vi "heterochromaticFlicker_digitalIN.vi"() -> ()   [LabVIEW 2011]
uses:
  <vilib>/LabVIEW Interface for Arduino/Type Defs/Pin Mode.ctl
  <vilib>/LabVIEW Interface for Arduino/LabVIEW Interface for Arduino.lvlib
panel:
  out "BUTTON":bool
  out "Joy DOWN":bool
  out "Joy UP":bool
  in  "Button Pin":u8=2
  in  "Joy DOWN Pin":u8=2
  in  "Joy UP Pin":u8=2
  in  "Stop":bool
  out "Debug \ninner i\n(which of the\nlights to be flashed)":i32
  out "Debug \nouter i\n(how many \ncycles passed)":i32
  in  "Duty Cycle 410nm 3":u8(slide) step=1 scale=0.0..255.0
  in  "Pin 560nm":dbl=2.0
  in  "Pin 410nm":dbl=2.0
  out "Flicker period [ms]":dbl=500.0
  in  "Flicker Freq [Hz]":dbl=2.0 min=0.2 max=100.0 step=0.1
  in  "Duty Cycle 410nm":u8(slide) step=1 scale=0.0..255.0
  in  "Duty Cycle 560nm":u8(slide) step=1 scale=0.0..255.0
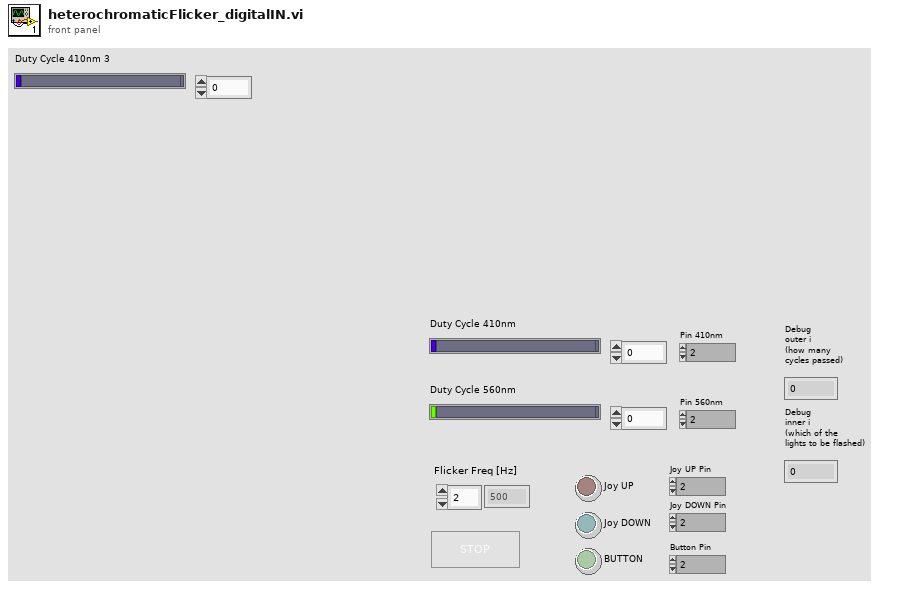
[diagram p1: front panel]
types:
  T1 = typedef "LabVIEW Interface for Arduino.lvlib/Arduino Resource.ctl" = cluster{"VISA resource":refnum<visa-resource-name>, "Board Type":T2, "Connection Type":enum8{"USB / Serial"}, "Bytes Per Packet (15)":u8}
  T2 = typedef "LabVIEW Interface for Arduino.lvlib/Board Type.ctl" = enum16{"Uno", "Dimuelanove w/Atmega 328", "Mega 2560"}
  T3 = typedef "LabVIEW Interface for Arduino.lvlib/Pin Mode.ctl" = enum8{"Input", "Output"}
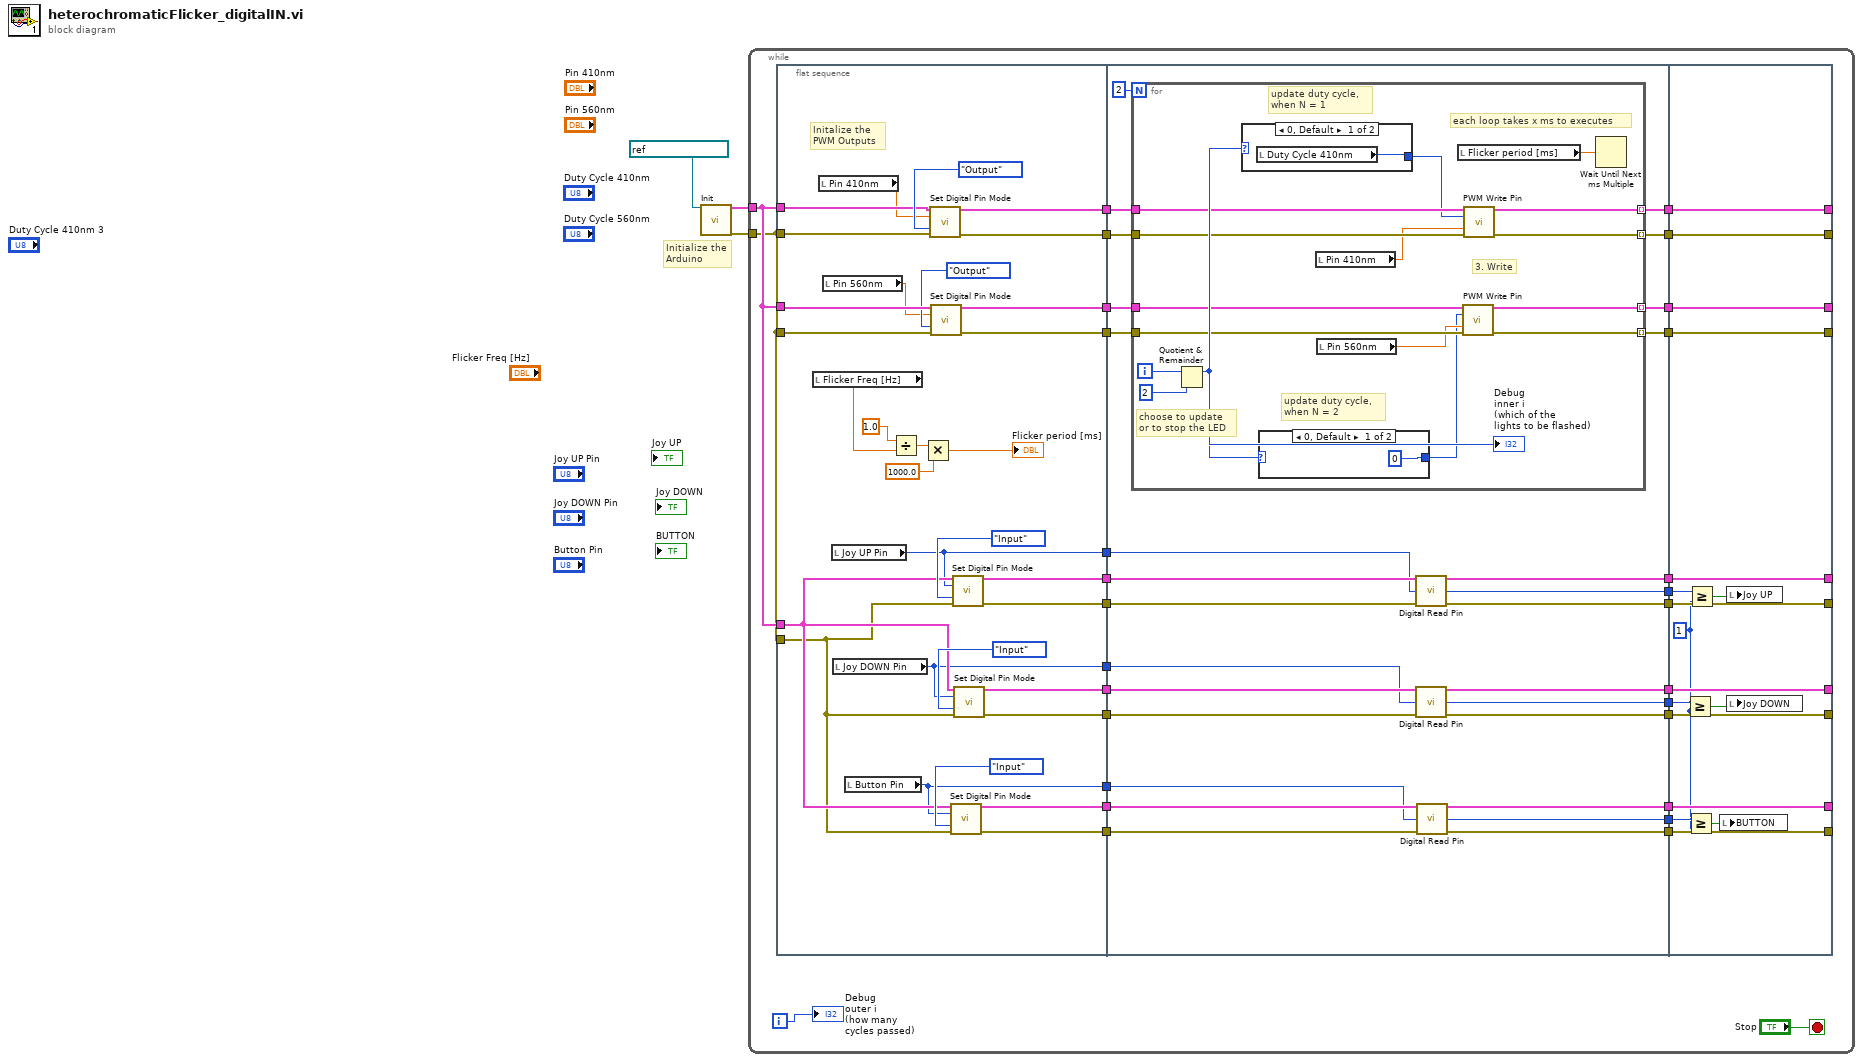
[diagram p0: block diagram]
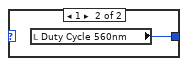
[diagram p2: hidden frame]
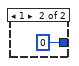
[diagram p3: hidden frame]
diagram:
  # "Initialize the\nArduino"
  n1 = call <vilib>:"Init.vi"("VISA resource"=refnum<visa-resource-name> "ASRL1::INSTR") -> ("Arduino Resource"=w3:T1, "error out"=w2:errorcluster)  [unwired: 17 in]
  n2 = while {
    tunnel: w3 -> [w23]
    tunnel: w2 -> [w22]
    i -> [w28]
    stop <- "Stop" stop-if-true
    n3 = flat-sequence {
      tunnel: w23 -> [w63]
      tunnel: w22 -> [w62]
      tunnel: w23 -> [w61]
      tunnel: w22 -> [w60]
      tunnel: [w56] -> w33
      tunnel: [w55] -> w32
      tunnel: [w54] -> w31
      tunnel: [w53] -> w30
      tunnel: w23 -> [w44]
      tunnel: w22 -> [w43]
      tunnel: [w42] -> w21
      tunnel: [w41] -> w20
      tunnel: [w40] -> w19
      tunnel: [w39] -> w18
      tunnel: [w38] -> w17
      tunnel: [w37] -> w16
      tunnel: [w36] -> w15
      tunnel: [w35] -> w14
      tunnel: [w34] -> w13
      tunnel: w33 -> [w90]
      tunnel: w32 -> [w89]
      tunnel: w31 -> [w88]
      tunnel: w30 -> [w87]
      tunnel: [w86] -> w27
      tunnel: [w85] -> w26
      tunnel: [w84] -> w25
      tunnel: [w83] -> w24
      tunnel: w21 -> [w82]
      tunnel: w20 -> [w81]
      tunnel: w19 -> [w80]
      tunnel: w18 -> [w79]
      tunnel: w17 -> [w78]
      tunnel: w16 -> [w77]
      tunnel: w15 -> [w76]
      tunnel: w14 -> [w75]
      tunnel: w13 -> [w74]
      tunnel: [w73] -> w12
      tunnel: [w72] -> w11
      tunnel: [w71] -> w10
      tunnel: [w70] -> w9
      tunnel: [w69] -> w8
      tunnel: [w68] -> w7
      tunnel: [w67] -> w6
      tunnel: [w66] -> w5
      tunnel: [w65] -> w4
      tunnel: [w125] -> _
      tunnel: [w126] -> _
      tunnel: [w127] -> _
      tunnel: [w128] -> _
      tunnel: w27 -> [w128]
      tunnel: w26 -> [w127]
      tunnel: w25 -> [w126]
      tunnel: w24 -> [w125]
      tunnel: [w124] -> _
      tunnel: w12 -> [w124]
      tunnel: [w123] -> _
      tunnel: w11 -> [w123]
      tunnel: [w122] -> _
      tunnel: w10 -> [w122]
      tunnel: [w121] -> _
      tunnel: w9 -> [w121]
      tunnel: [w120] -> _
      tunnel: w8 -> [w120]
      tunnel: [w119] -> _
      tunnel: w7 -> [w119]
      tunnel: w6 -> [w117]
      tunnel: w5 -> [w116]
      tunnel: w4 -> [w118]
      frame #0 {
        # "Initalize the \nPWM Outputs"
        n4 = local read "Flicker Freq [Hz]"() -> (w48:dbl)
        n5 = local read "Pin 410nm"() -> (w57:dbl)
        n6 = local read "Pin 560nm"() -> (w58:dbl)
        n7 = local read "Joy UP Pin"() -> (w34:u8)
        n8 = local read "Joy DOWN Pin"() -> (w35:u8)
        n9 = local read "Button Pin"() -> (w36:u8)
        n10 = Divide(x=1.0, y=w48) -> (x/y=w50:dbl)
        n11 = Multiply(x=w50, y=1000.0) -> (x*y=→"Flicker period [ms]":dbl)
        n12 = call <vilib>:"Set Digital Pin Mode.vi"("Arduino Resource"=w63, "Digital I/O Pin"=w57, "Pin Mode (Input)"=Pin_Mode."Output", "error in"=w62) -> ("Arduino Resource"=w54:T1, "error out"=w53:errorcluster)  [unwired: 10 in]
        n13 = call <vilib>:"Set Digital Pin Mode.vi"("Arduino Resource"=w61, "Digital I/O Pin"=w58, "Pin Mode (Input)"=Pin_Mode."Output", "error in"=w60) -> ("Arduino Resource"=w56:T1, "error out"=w55:errorcluster)  [unwired: 10 in]
        n14 = call <vilib>:"Set Digital Pin Mode.vi"("Arduino Resource"=w44, "Digital I/O Pin"=w36, "Pin Mode (Input)"=Pin_Mode."Input", "error in"=w43) -> ("Arduino Resource"=w38:T1, "error out"=w37:errorcluster)  [unwired: 10 in]
        n15 = call <vilib>:"Set Digital Pin Mode.vi"("Arduino Resource"=w44, "Digital I/O Pin"=w34, "Pin Mode (Input)"=Pin_Mode."Input", "error in"=w43) -> ("Arduino Resource"=w42:T1, "error out"=w41:errorcluster)  [unwired: 10 in]
        n16 = call <vilib>:"Set Digital Pin Mode.vi"("Arduino Resource"=w44, "Digital I/O Pin"=w35, "Pin Mode (Input)"=Pin_Mode."Input", "error in"=w43) -> ("Arduino Resource"=w40:T1, "error out"=w39:errorcluster)  [unwired: 10 in]
      }
      frame #1 {
        n17 = for {
          N: 2 -> [_]
          tunnel: w90 -> [w103]
          tunnel: w89 -> [w102]
          tunnel: w88 -> [w101]
          tunnel: w87 -> [w100]
          tunnel: [w99] -> w83 mode=indexing
          tunnel: [w98] -> w86 mode=indexing
          tunnel: [w97] -> w85 mode=indexing
          tunnel: [w96] -> w84 mode=indexing
          i -> [w105]
          # "update duty cycle, \nwhen N = 2"
          # "update duty cycle, \nwhen N = 1"
          # "each loop takes x ms to executes"
          # "3. Write"
          # "choose to update \nor to stop the LED"
          n18 = Quotient & Remainder(x=w105, y=2) -> (x-y*floor(x/y)=w104:i32)  [unwired: 1 out]
          n19 = case shown="0, Default" w104 {
            tunnel: [w110 u8 0 ("Duty Cycle")] -> w92
            frame 0, Default {
              n20 = local read "Duty Cycle 410nm"() -> (w110:u8)
            }
            frame 1 {
            }
          }
          n21 = case shown="0, Default" w104 {
            tunnel: [u8 0 ("Duty Cycle") w109] -> w94
            frame 0, Default {
            }
            frame 1 {
              n22 = local read "Duty Cycle 560nm"() -> (w109:u8)
            }
          }
          n23 = local read "Pin 410nm"() -> (w93:dbl)
          n24 = local read "Pin 560nm"() -> (w95:dbl)
          n25 = local read "Flicker period [ms]"() -> (w107:dbl)
          n26 = call <vilib>:"PWM Write Pin.vi"("Arduino Resource"=w103, "Duty Cycle (0 - 255)"=w94, "PWM Pin (3)"=w95, "error in"=w102) -> ("Arduino Resource"=w98:T1, "error out"=w97:errorcluster)  [unwired: 10 in]
          n27 = call <vilib>:"PWM Write Pin.vi"("Arduino Resource"=w101, "Duty Cycle (0 - 255)"=w92, "PWM Pin (3)"=w93, "error in"=w100) -> ("Arduino Resource"=w99:T1, "error out"=w96:errorcluster)  [unwired: 10 in]
          n28 = Wait Until Next ms Multiple(millisecond multiple=w107) -> ()  [unwired: 1 out]
          "Debug \ninner i\n(which of the\nlights to be flashed)" <- w105
        }
        n29 = call <vilib>:"Digital Read Pin.vi"("Arduino Resource"=w82, "Digital I/O Pin (0)"=w74, "error in"=w81) -> ("Arduino Resource"=w73:T1, "Value"=w65:u8, "error out"=w72:errorcluster)  [unwired: 10 in]
        n30 = call <vilib>:"Digital Read Pin.vi"("Arduino Resource"=w80, "Digital I/O Pin (0)"=w75, "error in"=w79) -> ("Arduino Resource"=w71:T1, "Value"=w66:u8, "error out"=w70:errorcluster)  [unwired: 10 in]
        n31 = call <vilib>:"Digital Read Pin.vi"("Arduino Resource"=w78, "Digital I/O Pin (0)"=w76, "error in"=w77) -> ("Arduino Resource"=w69:T1, "Value"=w67:u8, "error out"=w68:errorcluster)  [unwired: 10 in]
      }
      frame #2 {
        w115 = u8 1 ("y")
        n32 = Greater Or Equal?(x=w116, y=w115) -> (x >= y?=w114:bool)
        n33 = Greater Or Equal?(x=w117, y=w115) -> (x >= y?=w112:bool)
        n34 = Greater Or Equal?(x=w118, y=w115) -> (x >= y?=w113:bool)
        n35 = local write "BUTTON"(w112) -> ()
        n36 = local write "Joy UP"(w113) -> ()
        n37 = local write "Joy DOWN"(w114) -> ()
      }
    }
    "Debug \nouter i\n(how many \ncycles passed)" <- w28
  }
